vi "Joystick.vi"   [LabVIEW 2018]
uses:
  <vilib>/Rock Robotics/WPI/Joystick/WPI_JoystickDeviceEnum.ctl
  Type Defs/Read Write.ctl
types:
  T1 = typedef "WPI_JoystickDeviceEnum.ctl" = enum16{"USB 0", "USB 1", "USB 2", "USB 3", "USB 4", "USB 5"}
  T2 = typedef "WPI_JoystickDevRef.ctl" = cluster{"Device":T1}
  T3 = typedef "Read Write.ctl" = enum16{"Read", "Write"}
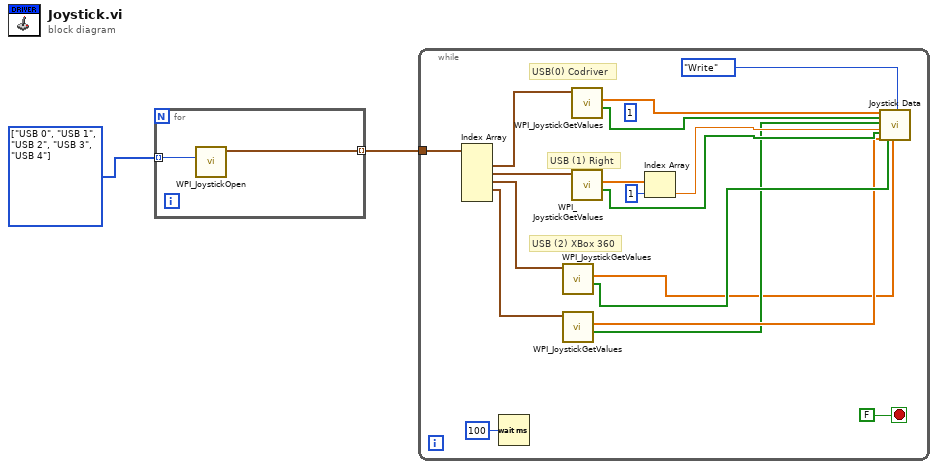
[diagram p0: block diagram]
diagram:
  w2 = T1[] [enum."USB 0", enum."USB 1", enum."USB 2", enum."USB 3", enum."USB 4"] items=["USB 0", "USB 1", "USB 2", "USB 3", "USB 4", "USB 5"]
  n1 = for {
    tunnel: w2 -> [w4] mode=indexing
    tunnel: [w3] -> w1 mode=indexing
    n2 = call <vilib>:"WPI_JoystickOpen.vi"("JoystickDevice"=w4) -> ("JoystickDevRef"=w3:T2)  [unwired: 10 in]
  }
  n3 = while {
    tunnel: w1 -> [w22]
    stop <- FALSE stop-if-true
    (unwired) 1 ("index")
    # "USB (2) XBox 360"
    # "USB (1) Right"
    # "USB(0) Codriver"
    n4 = Index Array(array=w22) -> (element #1=w21:T2, element #2=w20:T2, element #3=w19:T2, element #4=w5:T2)  [unwired: 5 in, 1 out]
    n5 = Wait (ms)(milliseconds to wait=u32 100) -> ()  [unwired: 1 out]
    n6 = call <vilib>:"WPI_JoystickGetValues.vi"("JoystickDevRef"=w19) -> ("Buttons"=w13:bool[], "Axes"=w7:dbl[])  [unwired: 6 in, 3 out]
    n7 = call <vilib>:"WPI_JoystickGetValues.vi"("JoystickDevRef"=w5) -> ("Buttons"=w8:bool[], "Axes"=w9:dbl[])  [unwired: 6 in, 3 out]
    n8 = call <vilib>:"WPI_JoystickGetValues.vi"("JoystickDevRef"=w21) -> ("Buttons"=w12:bool[], "Axes"=w6:dbl[])  [unwired: 6 in, 3 out]
    n9 = call <vilib>:"WPI_JoystickGetValues.vi"("JoystickDevRef"=w20) -> ("Buttons"=w10:bool[], "Axes"=w18:dbl[])  [unwired: 6 in, 3 out]
    n10 = Index Array(array=w18, index=1) -> (element=w11:dbl)
    n11 = call "Joystick Data.vi"("Joystick codrive in"=w6, "Joystick Button in"=w12, "Xbox One In"=w8, "Right Joystick In"=w11, "Right Buttons In"=w10, "Xbox One Joy In"=w9, "Xbox 360 in"=w13, "Xbox 360 Joy In"=w7, "Read/Write"=Read_Write."Write") -> ()  [unwired: 3 in, 8 out]
  }
